vi "Fetch Multi-point.vi"(8 "error in (no error)":errorcluster, 11 "NI DMM in":refnum<class "NI DMM.lvclass">) -> (0 "error out":errorcluster, 2 "Data":variant, 3 "NI DMM out":refnum<class "NI DMM.lvclass">)   [LabVIEW 2020, in "NI DMM.lvlib" / "NI DMM.lvclass"]
uses:
  NI DMM.lvclass
  NI DMM.lvclass/NI DMM.ctl
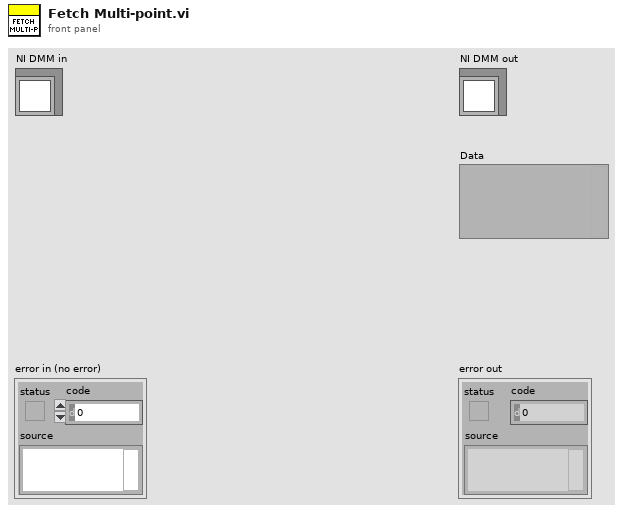
[diagram p1: front panel]
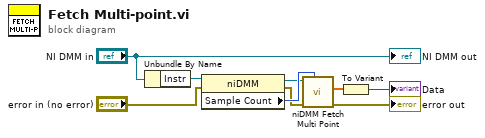
[diagram p0: block diagram]
diagram:
  n1 = Unbundle By Name("NI DMM in") -> ("Instr"=w6:refnum<k15>)
  n2 = property class="niDMM"(reference=w6, error in="error in (no error)") -> (reference out=w3:refnum<k15>, error out=w2:errorcluster, "Sample Count"=w4:i32)
  n3 = call <instrlib>:"niDMM Fetch Multi Point.vi"("Number to Fetch"=w4, "error in (no error)"=w2, "instrument handle"=w3) -> ("error out"=→"error out":errorcluster, "Measurements"=w8:dbl[])  [unwired: 5 in, 2 out]
  n4 = To Variant(anything=w8) -> (Variant=→"Data":variant)
  "NI DMM out" <- "NI DMM in"
